vi "Registry Monitor.vi"() -> ()   [LabVIEW 2013]
uses:
  src/SMO/Typedefs/SMOState --Enum.ctl
  src/Registry/Registry-SMO.lvclass
  src/SMO/SMO.lvclass
panel:
  in  "Check Context":bool
  out "output cluster":errorcluster
  in  "Registered SMOs":i32(listbox)
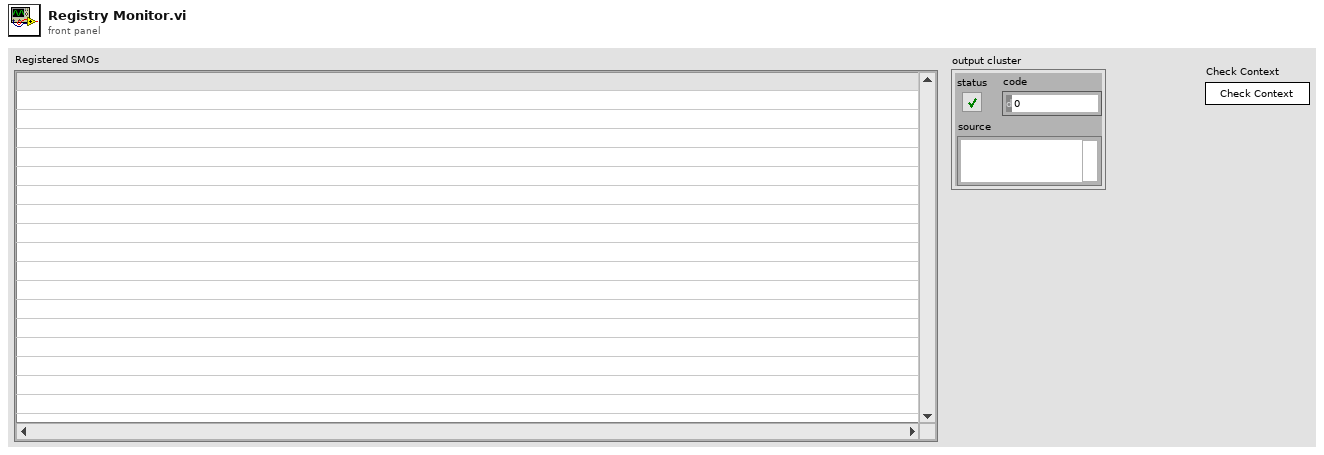
[diagram p1: front panel]
types:
  T1 = enum32{"invalid app kind", "Development System", "Run Time System", "Student Edition", "Embedded LabVIEW", "Evaluation", "Custom"}
  T2 = enum32{"Invalid", "Standard", "Closed", "Hidden", "Minimized", "Maximized"}
  T3 = cluster{"Core":cluster{"Current VI Reference":refnum<vi>, "Close Panel on Exit?":bool}, "Your Boolean data":bool, "Your string data":string}
  T4 = cluster{"Current VI Reference":refnum<vi>, "Close Panel on Exit?":bool}
  T5 = typedef "Registry-SMO.lvclass/PublicRegistryEvents--Cluster.ctl" = cluster{"Register Event":refnum<user-event>, "Unregister Event":refnum<user-event>}
  T6 = typedef "SMO.lvclass/Public Events.ctl" = cluster{"Error":refnum<user-event>, "State":refnum<user-event>}
  T7 = typedef "SMO.lvclass/SMOState --Enum.ctl" = enum16{"unknown", "Created", "Started", "Stopped"}
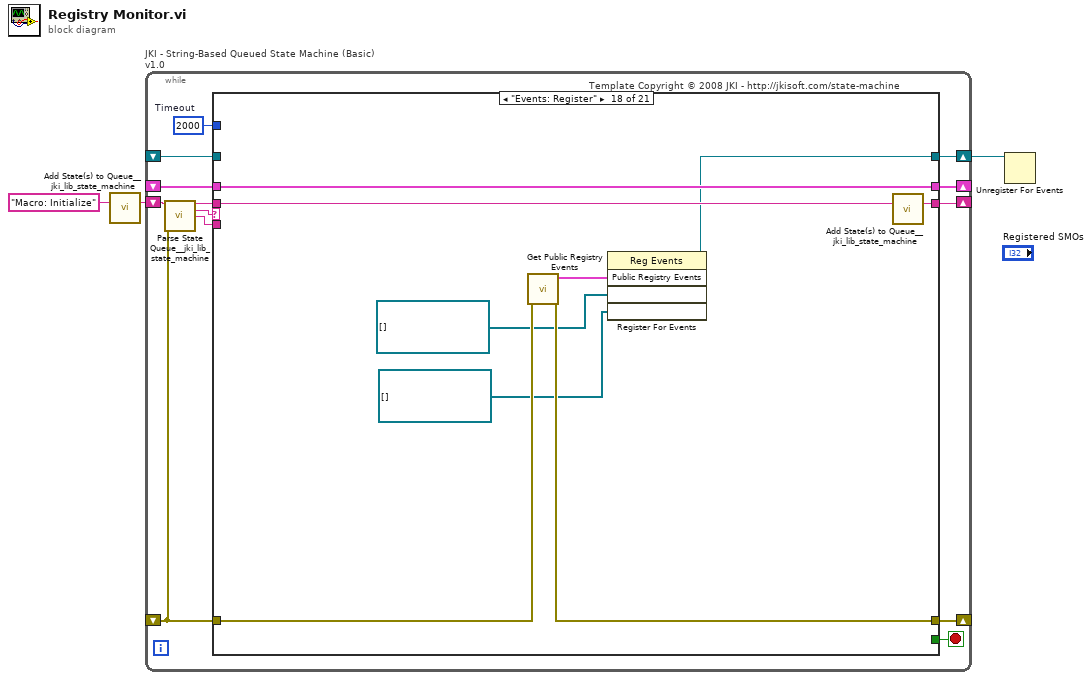
[diagram p0: block diagram]
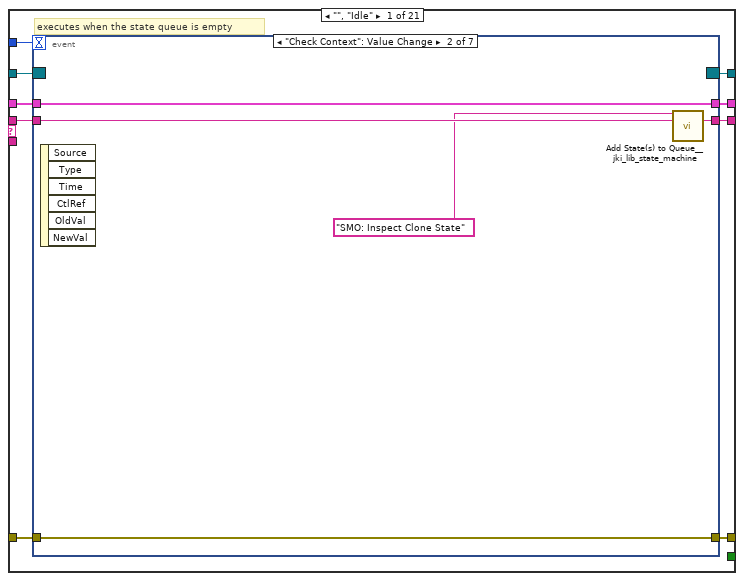
[diagram p2: hidden frame]
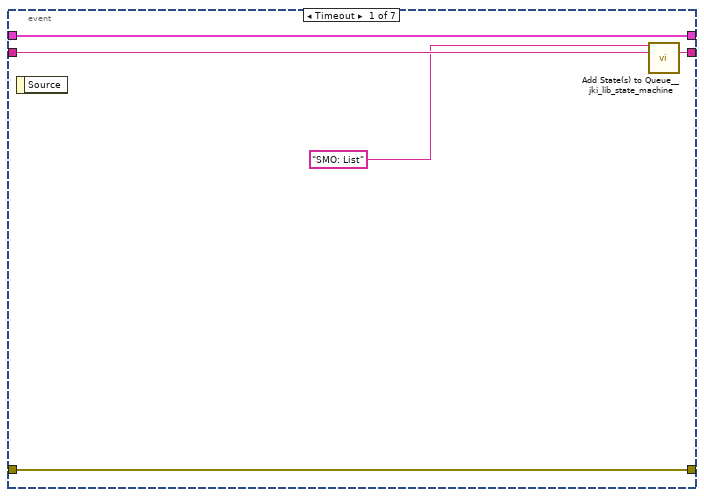
[diagram p3: hidden frame]
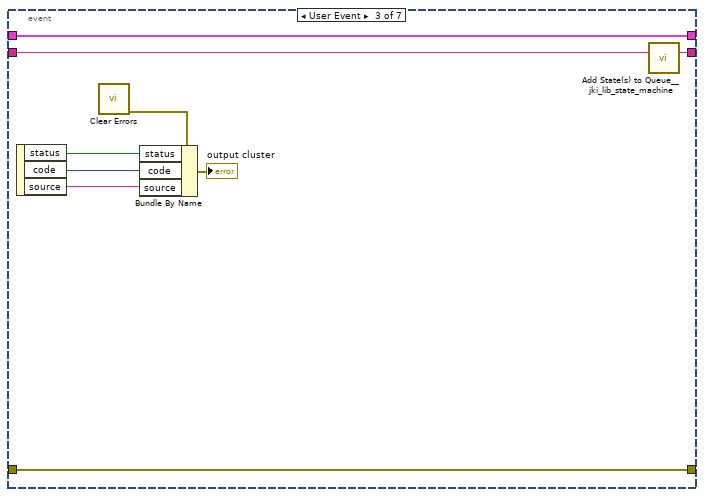
[diagram p4: hidden frame]
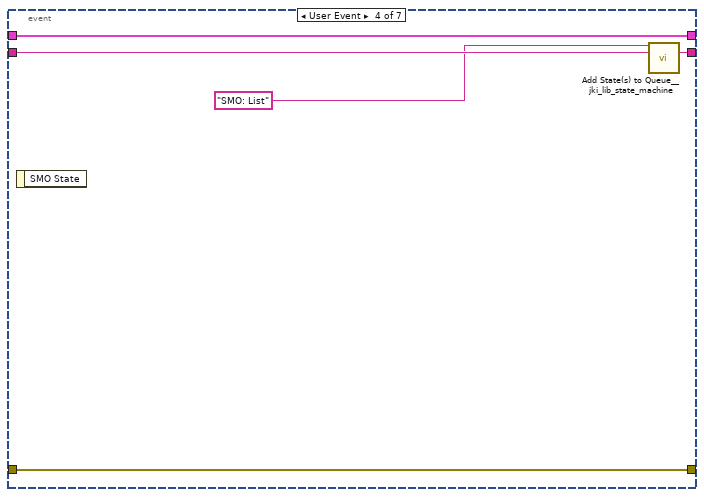
[diagram p5: hidden frame]
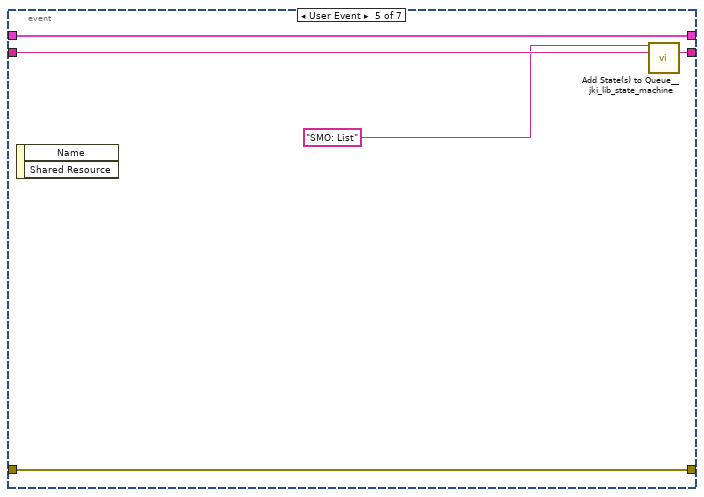
[diagram p6: hidden frame]
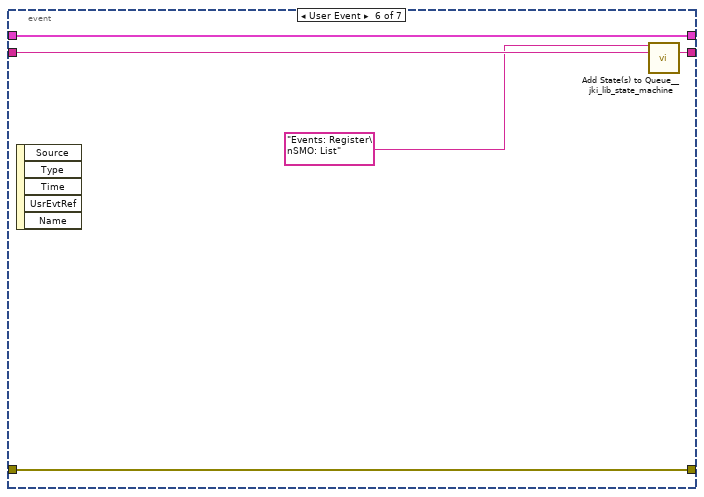
[diagram p7: hidden frame]
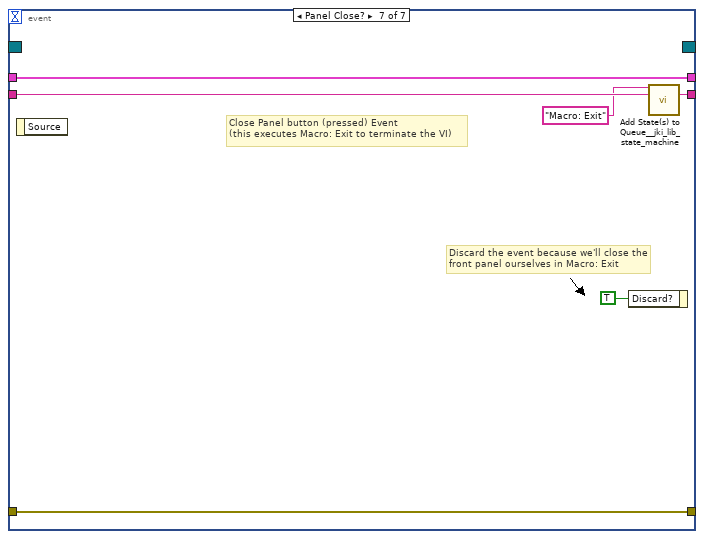
[diagram p8: hidden frame]
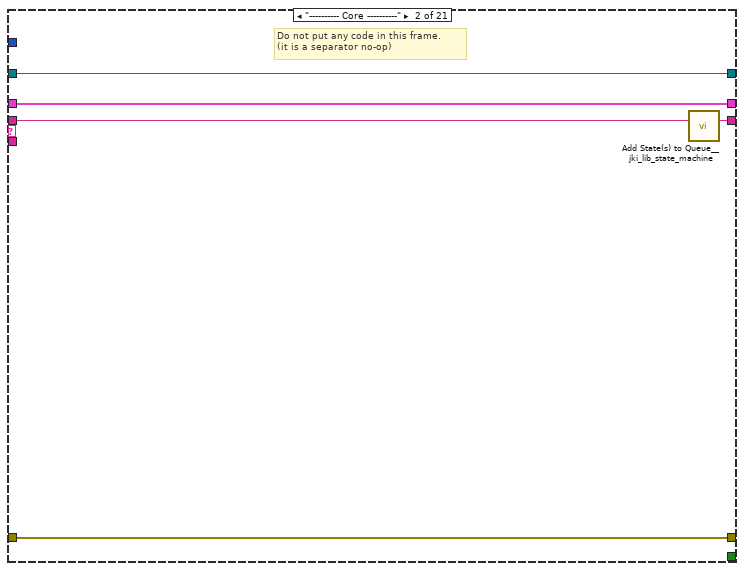
[diagram p9: hidden frame]
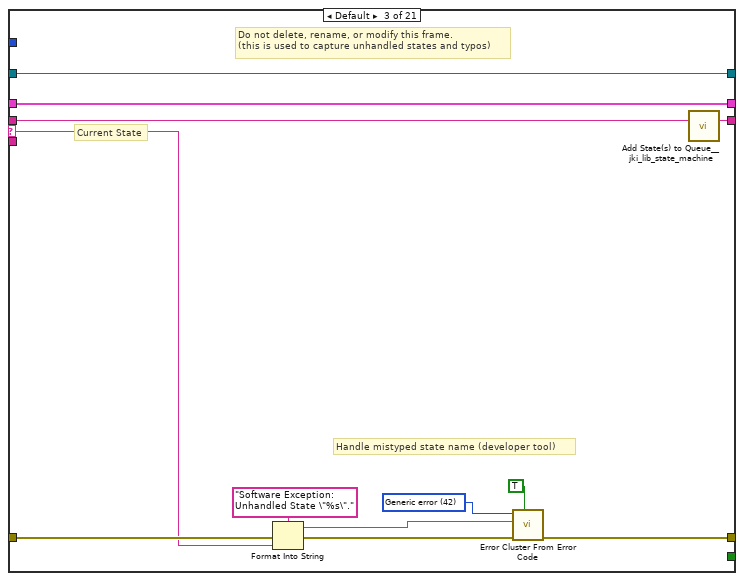
[diagram p10: hidden frame]
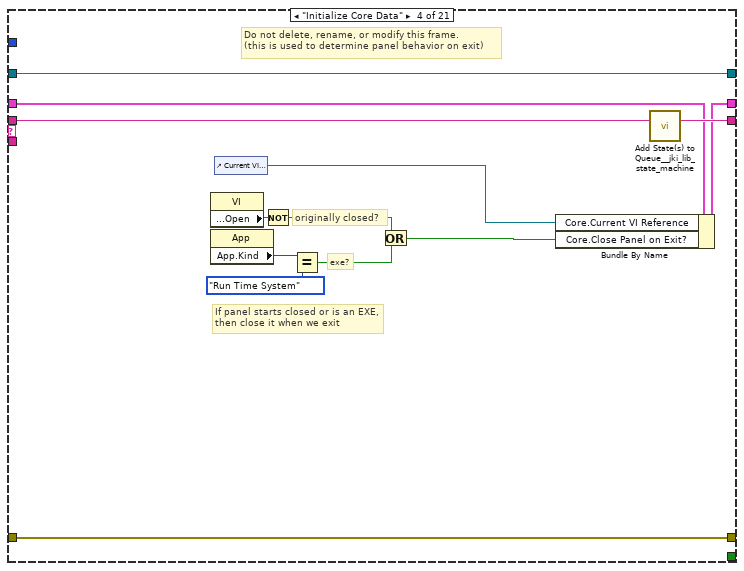
[diagram p11: hidden frame]
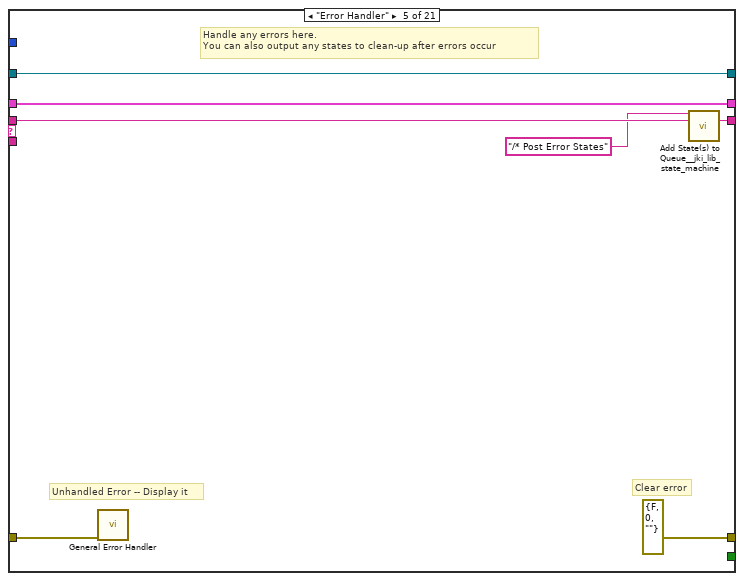
[diagram p12: hidden frame]
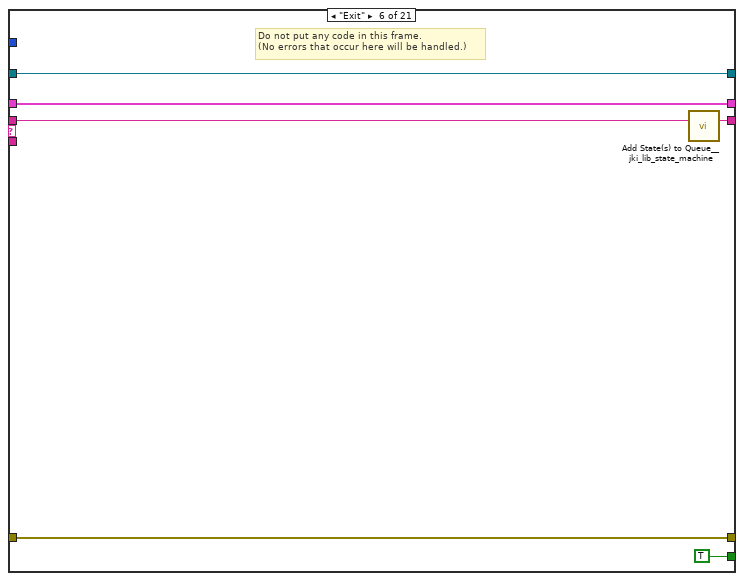
[diagram p13: hidden frame]
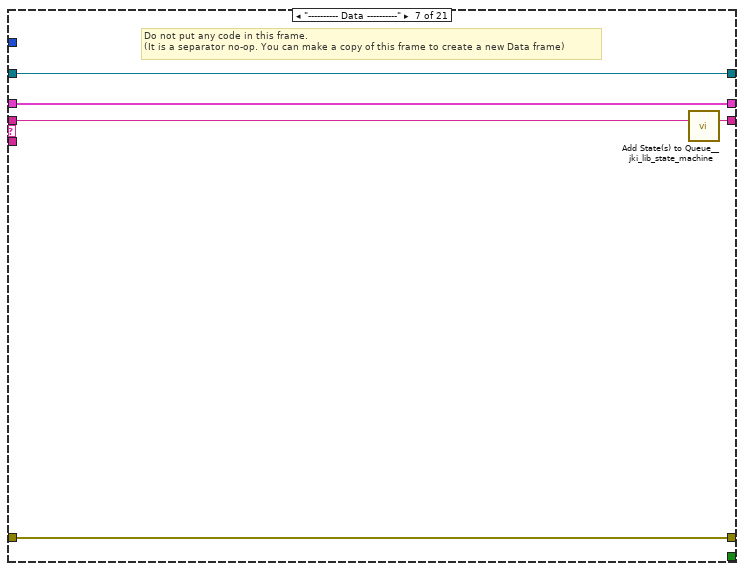
[diagram p14: hidden frame]
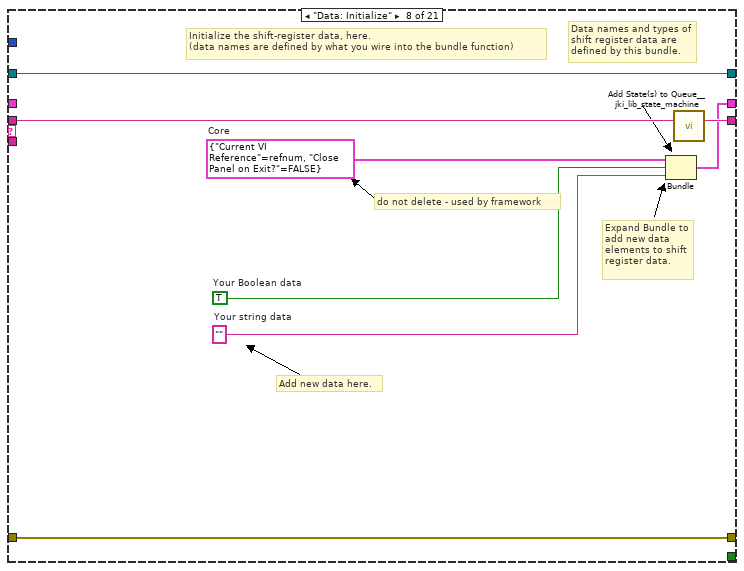
[diagram p15: hidden frame]
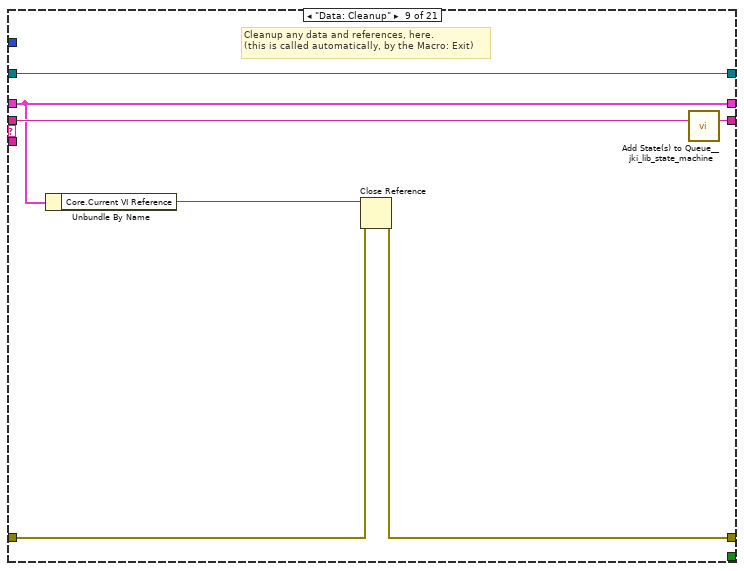
[diagram p16: hidden frame]
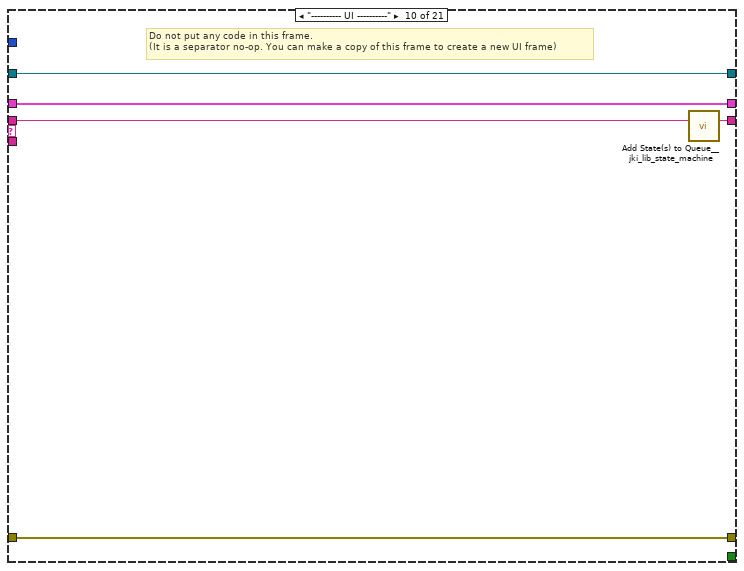
[diagram p17: hidden frame]
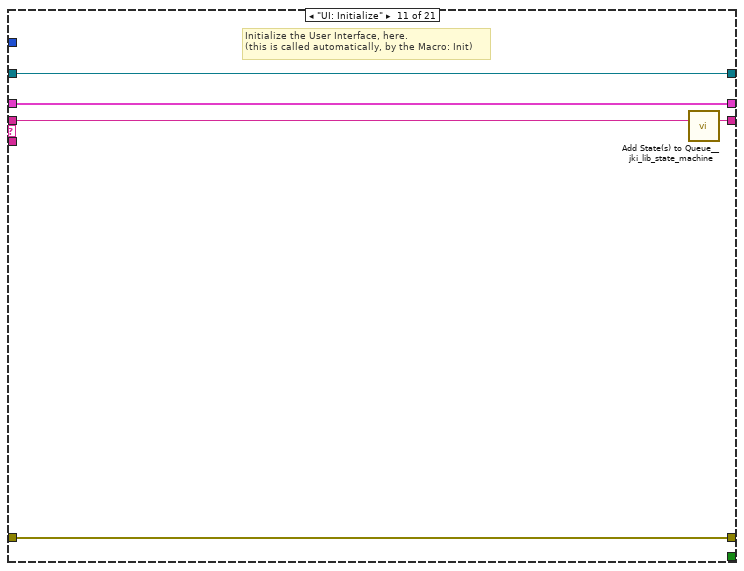
[diagram p18: hidden frame]
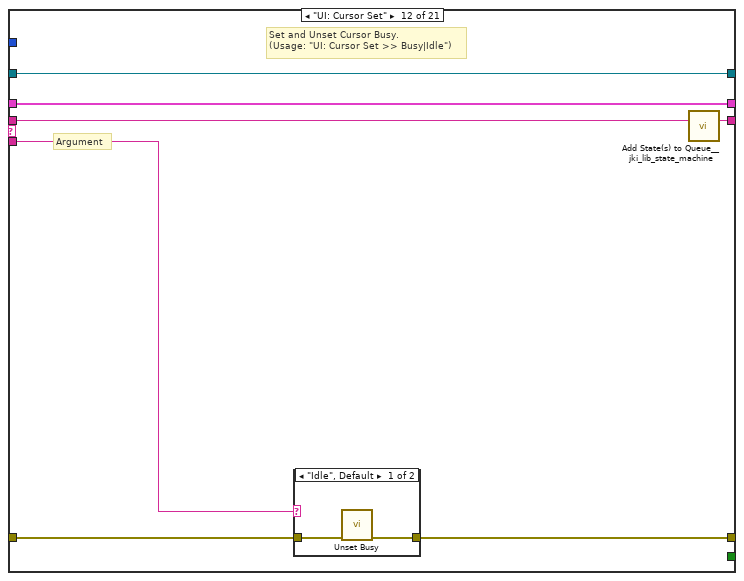
[diagram p19: hidden frame]
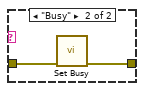
[diagram p20: hidden frame]
diagram:
  n1 = call <vilib>:"Add State(s) to Queue__jki_lib_state_machine.vi"("State(s) in (\"\")"="Macro: Initialize") -> ("States Out"=w3:string)  [unwired: 14 in]
  n2 = while "JKI - String-Based Queued State Machine (Basic) v1.0" {
    shift-right: [w9] -> _
    shift-left: _ -> [w8]
    shift-right: [w12] -> _
    shift-left: _ -> [w6]
    shift-right: [w11] -> _
    shift-left: w3 -> [w13]
    shift-right: [w4] -> w1
    shift-left: _ -> [w5]
    stop <- w10 stop-if-true
    w7 = 2000  # Timeout
    # "Template Copyright © 2008 JKI - http://jkisoft.com/state-machine"
    n3 = call <vilib>:"Parse State Queue__jki_lib_state_machine.vi"("State Queue"=w13, "Error In (no error)"=w6) -> ("Remaining States"=w15:string, "Current State"=w16:string, "Arguments"=w14:string)  [unwired: 11 in]
    n4 = case shown="\"Events: Register\"" w16 {
      selector: w16 -> [_ _ w72 _ _ _ _ _ _ _ _ _ _ _ _ _ _ _ _ _ _]
      tunnel: w15 -> [w25 w70 w76 w95 w102 w108 w113 w121 w128 w133 w138 w145 w157 w184 w190 w201 w206 w215 w220 w230 w253]
      tunnel: w14 -> [_ _ _ _ _ _ _ _ _ _ _ w140 w151 _ _ _ _ _ _ _ _]
      tunnel: w8 -> [w23 w67 w74 w86 w99 w106 w110 _ w123 w130 w136 w143 w153 w181 w187 w198 w203 w213 w217 w227 w250]
      tunnel: [w22 w68 w78 w92 errorcluster {"status"=FALSE, "code"=0, "source"=""} ("error out") w105 w111 w118 w124 w131 w135 w141 w154 w182 w188 w199 w204 w209 w218 w228 w251] -> w12
      tunnel: w6 -> [w21 w68 w77 w92 w98 w105 w111 w118 w125 w131 w135 w142 w155 w182 w188 w199 w204 w210 w218 w228 w251]
      tunnel: [w24 w69 w75 w94 w101 w107 w112 w120 w127 w132 w137 w144 w156 w183 w189 w200 w205 w214 w219 w229 w252] -> w11
      tunnel: [_ _ _ _ _ TRUE _ _ _ _ _ _ _ _ _ _ _ _ _ _ _] -> w10
      tunnel: [w20 w67 w74 w93 w99 w106 w110 w119 w123 w130 w136 w143 w153 w181 w187 w198 w203 w213 w217 w227 w250] -> w9
      tunnel: w7 -> [w19 _ _ _ _ _ _ _ _ _ _ _ _ _ _ _ _ _ _ _ _]
      tunnel: w5 -> [w18 w66 w71 w83 w96 w103 w109 w114 w122 w129 w134 w139 w150 w180 w185 w191 w202 _ w216 w224 w249]
      tunnel: [w17 w66 w71 w83 w96 w103 w109 w114 w122 w129 w134 w139 w150 w180 w185 w191 w202 w211 w216 w223 w249] -> w4
      frame "", "Idle" {
        # "executes when the state queue is empty"
        n5 = event shown="[1] \"Check Context\": Value Change" {
          selector: w18 -> [_ _ _ _ _ _ _]
          dyn-events: [_ _ _ _ _ _ _] -> w17
          timeout: w19 -> [_ _ _ _ _ _ _]
          tunnel: w25 -> [w30 w35 w44 w49 w54 w59 w65]
          tunnel: [w29 w34 w43 w48 w53 w58 w64] -> w24
          tunnel: w23 -> [w27 w32 w41 w46 w51 w56 w62]
          tunnel: [w28 w33 w42 w47 w52 w57 w63] -> w22
          tunnel: w21 -> [w28 w33 w42 w47 w52 w57 w63]
          tunnel: [w27 w32 w41 w46 w51 w56 w62] -> w20
          event Timeout {
            n6 = event-data() -> ()  [unwired: 1 in, 1 out]
            n7 = call <vilib>:"Add State(s) to Queue__jki_lib_state_machine.vi"("State(s) in Front (\"\")"="SMO: List", "State(s) in (\"\")"=w30) -> ("States Out"=w29:string)  [unwired: 13 in]
          }
          event "Check Context": Value Change {
            n8 = event-data() -> ()  [unwired: 1 in, 6 out]
            n9 = call <vilib>:"Add State(s) to Queue__jki_lib_state_machine.vi"("State(s) in Front (\"\")"="SMO: Inspect Clone State", "State(s) in (\"\")"=w35) -> ("States Out"=w34:string)  [unwired: 13 in]
          }
          event User Event {
            n10 = event-data() -> ("status"=w39:bool, "code"=w38:i32, "source"=w37:string)  [unwired: 1 in]
            n11 = call <vilib>:"Clear Errors.vi"() -> ("error out"=w40:errorcluster)  [unwired: 7 in]
            n12 = Bundle By Name(cluster=w40, "status"=w39, "code"=w38, "source"=w37) -> (→"output cluster":errorcluster)
            n13 = call <vilib>:"Add State(s) to Queue__jki_lib_state_machine.vi"("State(s) in (\"\")"=w44) -> ("States Out"=w43:string)  [unwired: 14 in]
          }
          event User Event {
            n14 = event-data() -> ()  [unwired: 1 in, 1 out]
            n15 = call <vilib>:"Add State(s) to Queue__jki_lib_state_machine.vi"("State(s) in Front (\"\")"="SMO: List", "State(s) in (\"\")"=w49) -> ("States Out"=w48:string)  [unwired: 13 in]
          }
          event User Event {
            n16 = event-data() -> ()  [unwired: 1 in, 2 out]
            n17 = call <vilib>:"Add State(s) to Queue__jki_lib_state_machine.vi"("State(s) in Front (\"\")"="SMO: List", "State(s) in (\"\")"=w54) -> ("States Out"=w53:string)  [unwired: 13 in]
          }
          event User Event {
            n18 = event-data() -> ()  [unwired: 1 in, 5 out]
            n19 = call <vilib>:"Add State(s) to Queue__jki_lib_state_machine.vi"("State(s) in Front (\"\")"="Events: Register\nSMO: List", "State(s) in (\"\")"=w59) -> ("States Out"=w58:string)  [unwired: 13 in]
          }
          event Panel Close? {
            # "Discard the event because we'll close the front panel ourselves in Macro: Exit"
            # "Close Panel button (pressed) Event\n(this executes Macro: Exit to terminate the VI)"
            n20 = event-data() -> ()  [unwired: 1 in, 1 out]
            n21 = event-data("Discard?"=TRUE) -> ()  [unwired: 1 in, 1 out]
            n22 = call <vilib>:"Add State(s) to Queue__jki_lib_state_machine.vi"("State(s) in Front (\"\")"="Macro: Exit", "State(s) in (\"\")"=w65) -> ("States Out"=w64:string)  [unwired: 13 in]
          }
        }
      }
      frame "---------- Core ----------" {
        # "Do not put any code in this frame.\n(it is a separator no-op)"
        n23 = call <vilib>:"Add State(s) to Queue__jki_lib_state_machine.vi"("State(s) in (\"\")"=w70) -> ("States Out"=w69:string)  [unwired: 14 in]
      }
      frame Default {
        w81 = 42 items=["No error", "Argument error", "Memory is full", "Out of zone", "End of file", "File already open", "Generic file I/O error", "File not found", "File permission error", "Disk is full", "Duplicate path", "Too many files open", "System feature not enabled", "Resource file not found", "Cannot add resource", "Resource not found", "Image not found", "Image memory error", "Pen does not exist", "Config type invalid", "Config token not found", "Config parse error", "Config memory error", "Bad external code format", "Bad external code offset", "External code not present", "Null window", "Destroy window error", "Null menu", "Print aborted", "Bad print record", "Print driver error", "Windows error during printing", "Memory error during printing", "Print dialog error", "Generic print error", "Invalid device refnum", "Device not found", "Device parameter error", "Device unit error", "Cannot open device", "Device call aborted", "Generic error", "Cancelled by user", "Object ID too low", "Object ID too high", "Object not in heap", "Unknown heap", "Unknown object (invalid DefProc)", "Unknown object (DefProc not in table)", "Message out of range", "Invalid (null) method", "Unknown message", "Manager call not supported", "Bad address", "Network operation in progress", "Network operation timed out", "Connection is busy", "Network attribute not supported", "Network error", "Address in use", "System out of memory", "Connection aborted", "Connection refused", "Not connected", "Already connected", "Connection closed", "Initialization error (interapplication manager)", "Bad occurrence", "Wait on unbound occurrence handler", "Occurrence queue overflow", "Datalog type conflict", "Unused", "Unrecognized type (interapplication manager)", "Memory corrupt", "Failed to make temporary DLL", "Old CIN version", "Drag socket not found", "Failed to load drop-object", "Failed to register OLE object", "Failed to release OLE object", "Format specifier type mismatch", "Unknown format specifier", "Too few format specifiers", "Too many format specifiers", "Scan failed", "Newer CIN version", "Error converting to variant", "Runtime menu error", "Password tampered", "Variant attribute not found", "Incompatible variant data type", "Event data is not available", "Event Store is not present", "Occurrence is not found", "Event Queue is not created", "Event info is not available", "Refnum passed is NULL", "Error retrieving Class GUID", "Error retrieving CoClass GUID", "Error retrieving TypeLib GUID.", "Bad built application magic bytes.", "Specific driver is different from the specific driver associated with the Logical Name.", "There is no session opened to the class driver.", "Max Error", "MAX - Error with config objects", "MAX - Error loading configuration", "MAX - Group not supported"]
        # "Current State"
        # "Do not delete, rename, or modify this frame.\n(this is used to capture unhandled states and typos)"
        # "Handle mistyped state name (developer tool)"
        n24 = Format Into String(format string="Software Exception: Unhandled State \"%s\"." ("message"), error in=w77, w72) -> (resulting string=w80:string, error out=w79:errorcluster)  [unwired: 1 in]
        n25 = call <vilib>:"Error Cluster From Error Code.vi"("show call chain? (False)"=TRUE, "error in (no error)"=w79, "error message (\"\")"=w80, "error code (0)"=w81) -> ("error out"=w78:errorcluster)  [unwired: 5 in]
        n26 = call <vilib>:"Add State(s) to Queue__jki_lib_state_machine.vi"("State(s) in (\"\")"=w76) -> ("States Out"=w75:string)  [unwired: 14 in]
      }
      frame "Initialize Core Data" {
        # "Do not delete, rename, or modify this frame.\n(this is used to determine panel behavior on exit)"
        # "originally closed?"
        # "exe?"
        # "If panel starts closed or is an EXE, then close it when we exit"
        n27 = property class="VI"() -> ("Front Panel.Open"=w91:bool)  [unwired: 2 in, 2 out]
        n28 = property class="App"() -> ("App.Kind"=w90:T1)  [unwired: 2 in, 2 out]
        n29 = control-ref of="Current VI Reference"() -> (w84:refnum<vi>)
        n30 = Not(x=w91) -> (.not. x?=w88:bool)
        n31 = Equal?(x=w90, y=T1."Run Time System" ("Application:Kind")) -> (x = y?=w87:bool)
        n32 = Or(x=w88, y=w87) -> (x .or. y?=w85:bool)
        n33 = Bundle By Name(cluster=w86, "Core.Current VI Reference"=w84, "Core.Close Panel on Exit?"=w85) -> (w93:T3)
        n34 = call <vilib>:"Add State(s) to Queue__jki_lib_state_machine.vi"("State(s) in (\"\")"=w95) -> ("States Out"=w94:string)  [unwired: 14 in]
      }
      frame "Error Handler" {
        # "Unhandled Error -- Display it"
        # "Handle any errors here.\nYou can also output any states to clean-up after errors occur"
        # "Clear error"
        n35 = call <vilib>:"General Error Handler.vi"("error in (no error)"=w98) -> ()  [unwired: 10 in, 5 out]
        n36 = call <vilib>:"Add State(s) to Queue__jki_lib_state_machine.vi"("State(s) in Front (\"\")"="/* Post Error States", "State(s) in (\"\")"=w102) -> ("States Out"=w101:string)  [unwired: 13 in]
      }
      frame "Exit" {
        # "Do not put any code in this frame.\n(No errors that occur here will be handled.)"
        n37 = call <vilib>:"Add State(s) to Queue__jki_lib_state_machine.vi"("State(s) in (\"\")"=w108) -> ("States Out"=w107:string)  [unwired: 14 in]
      }
      frame "---------- Data ----------" {
        # "Do not put any code in this frame.\n(It is a separator no-op. You can make a copy of this frame to create a new Data frame)"
        n38 = call <vilib>:"Add State(s) to Queue__jki_lib_state_machine.vi"("State(s) in (\"\")"=w113) -> ("States Out"=w112:string)  [unwired: 14 in]
      }
      frame "Data: Initialize" {
        w115 = T4 {"Current VI Reference"=refnum, "Close Panel on Exit?"=FALSE}  # Core
        w117 = TRUE  # Your Boolean data
        w116 = ""  # Your string data
        # "do not delete - used by framework"
        # "Expand Bundle to add new data elements to shift register data."
        # "Add new data here."
        # "Data names and types of shift register data are defined by this bundle."
        # "Initialize the shift-register data, here.\n(data names are defined by what you wire into the bundle function)"
        n39 = Bundle("Core"=w115, "Your Boolean data"=w117, "Your string data"=w116) -> (w119:T3)  [unwired: 1 in]
        n40 = call <vilib>:"Add State(s) to Queue__jki_lib_state_machine.vi"("State(s) in (\"\")"=w121) -> ("States Out"=w120:string)  [unwired: 14 in]
      }
      frame "Data: Cleanup" {
        # "Cleanup any data and references, here.\n(this is called automatically, by the Macro: Exit)"
        n41 = Unbundle By Name(w123) -> ("Core.Current VI Reference"=w126:refnum<vi>)
        n42 = Close Reference(reference=w126, error in (no error)=w125) -> (error out=w124:errorcluster)
        n43 = call <vilib>:"Add State(s) to Queue__jki_lib_state_machine.vi"("State(s) in (\"\")"=w128) -> ("States Out"=w127:string)  [unwired: 14 in]
      }
      frame "---------- UI ----------" {
        # "Do not put any code in this frame.\n(It is a separator no-op. You can make a copy of this frame to create a new UI frame)"
        n44 = call <vilib>:"Add State(s) to Queue__jki_lib_state_machine.vi"("State(s) in (\"\")"=w133) -> ("States Out"=w132:string)  [unwired: 14 in]
      }
      frame "UI: Initialize" {
        # "Initialize the User Interface, here.\n(this is called automatically, by the Macro: Init)"
        n45 = call <vilib>:"Add State(s) to Queue__jki_lib_state_machine.vi"("State(s) in (\"\")"=w138) -> ("States Out"=w137:string)  [unwired: 14 in]
      }
      frame "UI: Cursor Set" {
        # "Argument"
        # "Set and Unset Cursor Busy.\n(Usage: \"UI: Cursor Set >> Busy|Idle\")"
        n46 = case shown="\"Idle\", Default" w140 {
          tunnel: w142 -> [w147 w149]
          tunnel: [w146 w148] -> w141
          frame "Idle", Default {
            n47 = call <vilib>:"Unset Busy.vi"("error in (no error)"=w147) -> ("error out"=w146:errorcluster)  [unwired: 10 in]
          }
          frame "Busy" {
            n48 = call <vilib>:"Set Busy.vi"("error in (no error)"=w149) -> ("error out"=w148:errorcluster)  [unwired: 9 in, 1 out]
          }
        }
        n49 = call <vilib>:"Add State(s) to Queue__jki_lib_state_machine.vi"("State(s) in (\"\")"=w145) -> ("States Out"=w144:string)  [unwired: 14 in]
      }
      frame "UI: Front Panel State" {
        # "Argument"
        # "Set Front Panel Open or Closed\n(Usage: \"UI: Front Panel State >> Open|Close\")"
        n50 = Unbundle By Name(w153) -> ("Core.Current VI Reference"=w152:refnum<vi>)
        n51 = case shown="\"Open\", Default" w151 {
          tunnel: w155 -> [w161 w174]
          tunnel: [w163 w175] -> w154
          tunnel: w152 -> [w162 w172]
          frame "Open", Default {
            n52 = property class="VI"(reference=w162, error in=w161) -> (reference out=w159:refnum<vi>, error out=w160:errorcluster, "Front Panel.Open"=w158:bool)
            n53 = case shown="False" w158 {
              tunnel: [w166 w169] -> w163
              tunnel: w160 -> [w165 w169]
              tunnel: w159 -> [w164 _]
              frame False {
                n54 = invoke class="VI" method="FP.Open"(reference=w164, error in=w165, "Activate"=TRUE, "State"=T2."Standard") -> (error out=w166:errorcluster)  [unwired: 1 in, 4 out]
              }
              frame True {
              }
            }
          }
          frame "Close" {
            n55 = property class="VI"(reference=w172, error in=w174) -> (reference out=w171:refnum<vi>, error out=w173:errorcluster, "Front Panel.Open"=w170:bool)
            n56 = case shown="True" w170 {
              tunnel: [w176 w179] -> w175
              tunnel: w173 -> [w176 w178]
              tunnel: w171 -> [_ w177]
              frame False {
              }
              frame True {
                n57 = invoke class="VI" method="FP.Close"(reference=w177, error in=w178) -> (error out=w179:errorcluster)  [unwired: 1 in, 2 out]
              }
            }
          }
        }
        n58 = call <vilib>:"Add State(s) to Queue__jki_lib_state_machine.vi"("State(s) in (\"\")"=w157) -> ("States Out"=w156:string)  [unwired: 14 in]
      }
      frame "---------- Macro ----------" {
        # "Do not put any code in this frame.\n(It is a separator no-op. You can make a copy of this frame to create a new Macro frame)"
        n59 = call <vilib>:"Add State(s) to Queue__jki_lib_state_machine.vi"("State(s) in (\"\")"=w184) -> ("States Out"=w183:string)  [unwired: 14 in]
      }
      frame "Macro: Initialize" {
        w186 = "Data: Initialize\nInitialize Core Data\nUI: Initialize\nUI: Front Panel State >> Open\nEvents: Register\nSMO: List"  # Data: Initialize Initialize Core Data UI: Initialize UI: Front Panel State >> Open Events: Register SMO: List
        # "Initialization Macro\n(This is called once, when the VI starts)"
        n60 = call <vilib>:"Add State(s) to Queue__jki_lib_state_machine.vi"("State(s) in Front (\"\")"=w186, "State(s) in (\"\")"=w190) -> ("States Out"=w189:string)  [unwired: 13 in]
      }
      frame "Macro: Exit" {
        # "Exit Macro\n(This is called once, when the VI exits)"
        n61 = Unbundle By Name(w198) -> ("Core.Close Panel on Exit?"=w197:bool)
        n62 = Select(t="UI: Front Panel State >> Close", s=w197, f="") -> (s? t:f=w194:string)
        n63 = call <vilib>:"Add State(s) to Queue__jki_lib_state_machine.vi"("State(s) in (\"\")"=w194, "State(s) at Back (\"\")"="Data: Cleanup\nExit") -> ("States Out"=w192:string)  [unwired: 13 in]
        n64 = call <vilib>:"Add State(s) to Queue__jki_lib_state_machine.vi"("State(s) in Front (\"\")"=w192, "State(s) in (\"\")"=w201) -> ("States Out"=w200:string)  [unwired: 13 in]
      }
      frame "---------- Events ----------" {
        n65 = call <vilib>:"Add State(s) to Queue__jki_lib_state_machine.vi"("State(s) in (\"\")"=w206) -> ("States Out"=w205:string)  [unwired: 14 in]
      }
      frame "Events: Register" {
        w207 = refnum<user-event>[] [] items=["unknown", "Created", "Started", "Stopped"]
        n66 = call "Get Public Registry Events.vi"("error in (no error)"=w210) -> ("error out"=w209:errorcluster, "Public Registry Events"=w212:T5)  [unwired: 9 in]
        n67 = register-events(w212, refnum<user-event>[] [], w207) -> (reference out=w211:refnum<event-registration>)  [unwired: 2 in, 1 out]
        n68 = call <vilib>:"Add State(s) to Queue__jki_lib_state_machine.vi"("State(s) in (\"\")"=w215) -> ("States Out"=w214:string)  [unwired: 14 in]
      }
      frame "---------- SMO ----------" {
        n69 = call <vilib>:"Add State(s) to Queue__jki_lib_state_machine.vi"("State(s) in (\"\")"=w220) -> ("States Out"=w219:string)  [unwired: 14 in]
      }
      frame "SMO: List" {
        n70 = call "List Subsystems.vi"() -> ("Subsystems"=w225:refnum<class "SMO.lvclass">[])  [unwired: 10 in, 1 out]
        n71 = for {
          tunnel: w225 -> [w235] mode=indexing
          tunnel: [w240] -> w226 mode=indexing
          tunnel: [w236] -> _ mode=indexing
          tunnel: [w232] -> w222 mode=indexing
          tunnel: [w231] -> w221 mode=indexing
          n72 = call "GetPublicEvents.vi"("SMO"=w235) -> ("Public Events"=w233:T6, "SMO out"=w234:refnum<class "SMO.lvclass">)  [unwired: 8 in, 1 out]
          n73 = Unbundle By Name(w233) -> ("Error"=w232:refnum<user-event>, "State"=w231:refnum<user-event>)
          n74 = call "Get Name.vi"("SMO"=w234) -> ("error out"=w239:errorcluster, "Name"=w244:string, "SMO out"=w248:refnum<class "SMO.lvclass">)  [unwired: 8 in]
          n75 = call "Get State.vi"("error in (no error)"=w239, "SMO"=w248) -> ("error out"=w238:errorcluster, "SMO State"=w245:T7, "SMO out"=w247:refnum<class "SMO.lvclass">)  [unwired: 7 in]
          n76 = Format Into String(w245) -> (resulting string=w243:string)  [unwired: 3 in, 1 out]
          n77 = call "Get GUID.vi"("error in (no error)"=w238, "SMO"=w247) -> ("error out"=w237:errorcluster, "GUID"=w241:string, "SMO out"=w246:refnum<class "SMO.lvclass">)  [unwired: 7 in]
          n78 = call "Get Qualified Name.vi"("error in (no error)"=w237, "SMO"=w246) -> ("error out"=w236:errorcluster, "Qualified Name"=w242:string)  [unwired: 7 in, 1 out]
          n79 = Build Array(w244, w243, w242, w241) -> (w240:string[])
        }
        n80 = register-events(reference=w224, w222, w221) -> (reference out=w223:refnum<event-registration>)  [unwired: 2 in, 1 out]
        n81 = property on="Registered SMOs" class="MCListbox (strict)"("ItemNames"=w226) -> ()  [unwired: 2 in, 2 out]
        n82 = call <vilib>:"Add State(s) to Queue__jki_lib_state_machine.vi"("State(s) in (\"\")"=w230) -> ("States Out"=w229:string)  [unwired: 14 in]
      }
      frame "SMO: Inspect Clone State" {
        n83 = property class="App" props=["App.AllVIs"]() -> ()  [unwired: 2 in, 3 out]
        n84 = call <vilib>:"Add State(s) to Queue__jki_lib_state_machine.vi"("State(s) in (\"\")"=w253) -> ("States Out"=w252:string)  [unwired: 14 in]
      }
    }
  }
  n85 = Unregister For Events(event registration refnum=w1) -> ()  [unwired: 1 in, 1 out]
